vi "Get QE.vi"(7 "QE":sgl, 9 "mode":u32, 10 "wavelength":sgl, 11 "sensor":string) -> (2 "function return":u32, 3 "sensor out":string, 5 "QE out":sgl)   [LabVIEW 2018, in "AndorSDK.lvlib"]
doc: "EXPNETTYPE unsigned int WINAPI GetQE(char * sensor, float wavelength, unsigned int mode, float * QE);"
uses:
  AndorSDK.lvlib
  ATMCD32D.dll
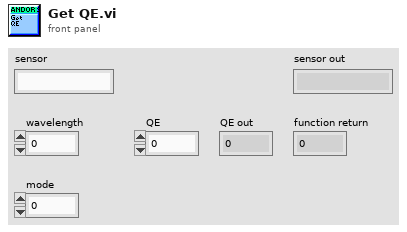
[diagram p1: front panel]
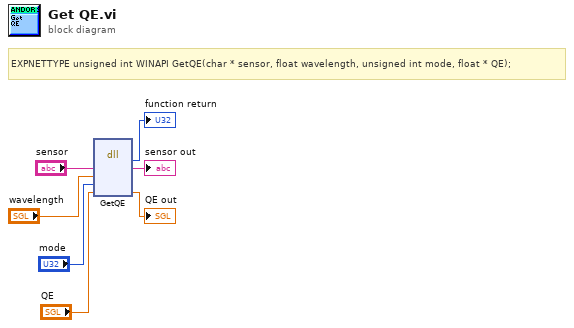
[diagram p0: block diagram]
diagram:
  # "EXPNETTYPE unsigned int WINAPI GetQE(char * sensor, float wavelength, unsigned int mode, float * QE);"
  n1 = dll-call lib="PTH2babs E\nPersönliches02 - Arbeit03-HiwijobsLabviewCodelibANDOR\tAndor SDK\nATMCD32D.*" fn="GetQE"("sensor"="sensor", "wavelength"="wavelength", "mode"="mode", "QE"="QE") -> (→"function return":u32, "sensor"=→"sensor out":string, "QE"=→"QE out":sgl)  [unwired: 5 in, 2 out]
